vi "자판기.vi"() -> ()   [LabVIEW 2011]
panel:
  in  "거스름돈 반환":bool
  out "거스름돈":i32 format="%d \\"
  in  "투입금액":i32 format="%d \\"
  in  "생수":bool
  in  "사이다":bool
  in  "콜라":bool
  in  "커피":bool
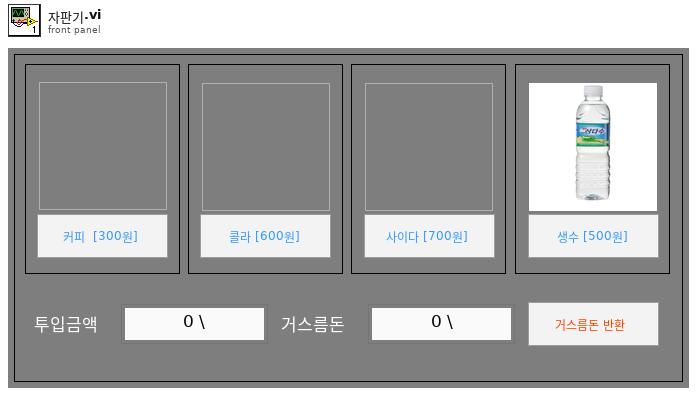
[diagram p1: front panel]
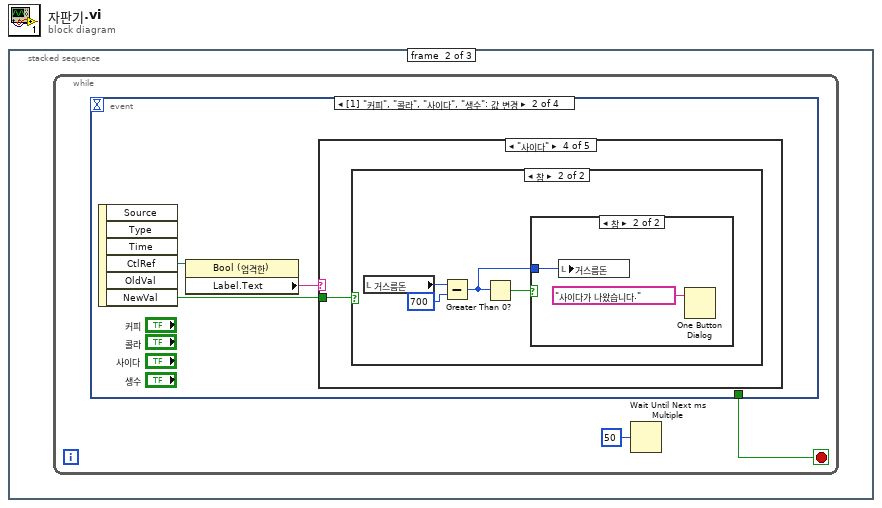
[diagram p0: block diagram]
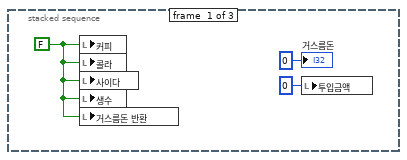
[diagram p2: hidden frame]
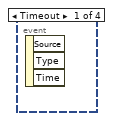
[diagram p3: hidden frame]
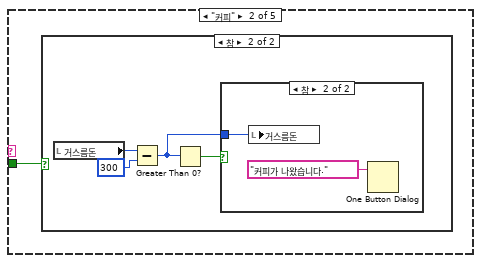
[diagram p5: hidden frame]
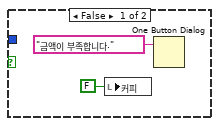
[diagram p7: hidden frame]
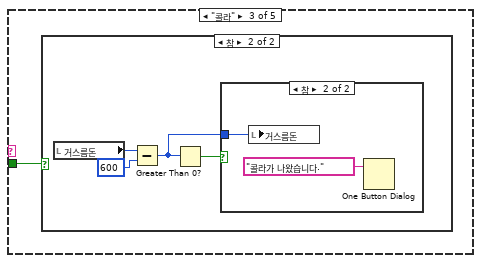
[diagram p8: hidden frame]
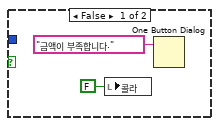
[diagram p10: hidden frame]
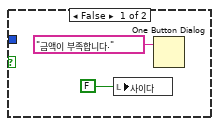
[diagram p12: hidden frame]
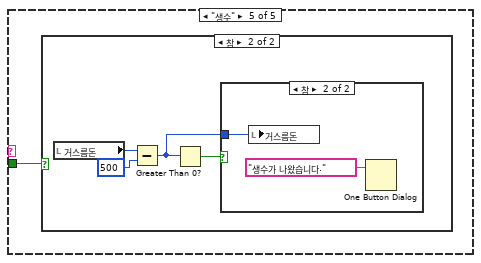
[diagram p13: hidden frame]
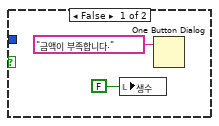
[diagram p15: hidden frame]
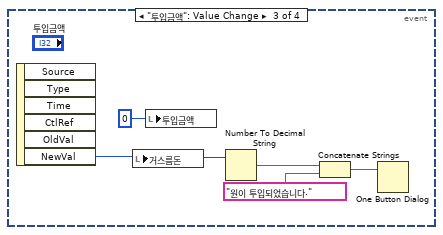
[diagram p16: hidden frame]
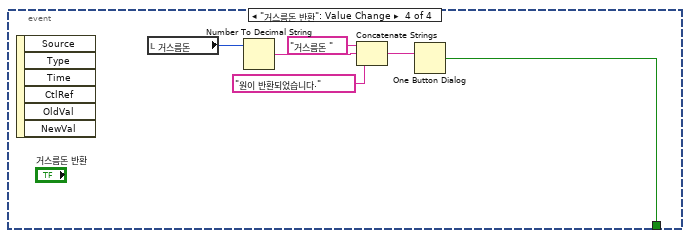
[diagram p17: hidden frame]
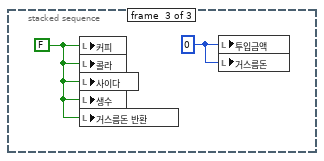
[diagram p18: hidden frame]
diagram:
  n1 = stacked-sequence {
    frame #0 {
      w3 = FALSE ("커피")
      n2 = local write "커피"(w3) -> ()
      n3 = local write "콜라"(w3) -> ()
      n4 = local write "사이다"(w3) -> ()
      n5 = local write "생수"(w3) -> ()
      n6 = local write "거스름돈 반환"(w3) -> ()
      n7 = local write "투입금액"(0 ("투입금액")) -> ()
      "거스름돈" <- 0 ("거스름돈")
    }
    frame #1 {
      n8 = while {
        stop <- w5 stop-if-true
        n9 = event shown="[1] \"커피\", \"콜라\", \"사이다\", \"생수\": 값 변경" {
          selector: _ -> [_ _ _ _]
          dyn-events: _ -> [_ _ _ _]
          timeout: _ -> [_ _ _ _]
          tunnel: [_ _ _ w50] -> w5
          event Timeout {
            n10 = event-data() -> ()  [unwired: 1 in, 3 out]
          }
          event "커피", "콜라", "사이다", "생수": Value Change {
            n11 = event-data() -> ("CtlRef"=w8:refnum<vi>, "NewVal"=w6:bool)  [unwired: 1 in, 4 out]
            n12 = property class="Bool (엄격한)"(reference=w8) -> ("Label.Text"=w7:string)  [unwired: 1 in, 2 out]
            n13 = case shown="\"사이다\"" w7 {
              tunnel: w6 -> [_ w9 w18 w27 w36]
              frame "거짓", Default {
              }
              frame "커피" {
                n14 = case shown="참" w9 {
                  frame False {
                  }
                  frame True {
                    n15 = local read "거스름돈"() -> (w11:i32)
                    n16 = Subtract(x=w11, y=300) -> (x-y=w10:i32)
                    n17 = Greater Than 0?(x=w10) -> (x > 0?=w12:bool)
                    n18 = case shown="참" w12 {
                      tunnel: w10 -> [_ w17]
                      frame False {
                        n19 = local write "커피"(FALSE ("커피")) -> ()
                        n20 = One Button Dialog(message="금액이 부족합니다." ("메시지")) -> ()  [unwired: 1 in, 1 out]
                      }
                      frame True {
                        n21 = local write "거스름돈"(w17) -> ()
                        n22 = One Button Dialog(message="커피가 나왔습니다." ("메시지")) -> ()  [unwired: 1 in, 1 out]
                      }
                    }
                  }
                }
              }
              frame "콜라" {
                n23 = case shown="참" w18 {
                  frame False {
                  }
                  frame True {
                    n24 = local read "거스름돈"() -> (w20:i32)
                    n25 = Subtract(x=w20, y=600) -> (x-y=w19:i32)
                    n26 = Greater Than 0?(x=w19) -> (x > 0?=w21:bool)
                    n27 = case shown="참" w21 {
                      tunnel: w19 -> [_ w26]
                      frame False {
                        n28 = local write "콜라"(FALSE ("커피")) -> ()
                        n29 = One Button Dialog(message="금액이 부족합니다." ("메시지")) -> ()  [unwired: 1 in, 1 out]
                      }
                      frame True {
                        n30 = local write "거스름돈"(w26) -> ()
                        n31 = One Button Dialog(message="콜라가 나왔습니다." ("메시지")) -> ()  [unwired: 1 in, 1 out]
                      }
                    }
                  }
                }
              }
              frame "사이다" {
                n32 = case shown="참" w27 {
                  frame False {
                  }
                  frame True {
                    n33 = local read "거스름돈"() -> (w29:i32)
                    n34 = Subtract(x=w29, y=700) -> (x-y=w28:i32)
                    n35 = Greater Than 0?(x=w28) -> (x > 0?=w30:bool)
                    n36 = case shown="참" w30 {
                      tunnel: w28 -> [_ w35]
                      frame False {
                        n37 = local write "사이다"(FALSE ("커피")) -> ()
                        n38 = One Button Dialog(message="금액이 부족합니다." ("메시지")) -> ()  [unwired: 1 in, 1 out]
                      }
                      frame True {
                        n39 = local write "거스름돈"(w35) -> ()
                        n40 = One Button Dialog(message="사이다가 나왔습니다." ("메시지")) -> ()  [unwired: 1 in, 1 out]
                      }
                    }
                  }
                }
              }
              frame "생수" {
                n41 = case shown="참" w36 {
                  frame False {
                  }
                  frame True {
                    n42 = local read "거스름돈"() -> (w38:i32)
                    n43 = Subtract(x=w38, y=500) -> (x-y=w37:i32)
                    n44 = Greater Than 0?(x=w37) -> (x > 0?=w39:bool)
                    n45 = case shown="참" w39 {
                      tunnel: w37 -> [_ w44]
                      frame False {
                        n46 = local write "생수"(FALSE ("커피")) -> ()
                        n47 = One Button Dialog(message="금액이 부족합니다." ("메시지")) -> ()  [unwired: 1 in, 1 out]
                      }
                      frame True {
                        n48 = local write "거스름돈"(w44) -> ()
                        n49 = One Button Dialog(message="생수가 나왔습니다." ("메시지")) -> ()  [unwired: 1 in, 1 out]
                      }
                    }
                  }
                }
              }
            }
          }
          event "투입금액": Value Change {
            n50 = event-data() -> ("NewVal"=w49:i32)  [unwired: 1 in, 5 out]
            n51 = local write "거스름돈"(w49) -> ()
            n52 = local write "투입금액"(0 ("투입금액")) -> ()
            n53 = Number To Decimal String(number=w49) -> (decimal integer string=w48:string)  [unwired: 1 in]
            n54 = Concatenate Strings(w48, "원이 투입되었습니다." ("문자열")) -> (w46:string)
            n55 = One Button Dialog(message=w46) -> ()  [unwired: 1 in, 1 out]
          }
          event "거스름돈 반환": Value Change {
            n56 = event-data() -> ()  [unwired: 1 in, 6 out]
            n57 = local read "거스름돈"() -> (w55:i32)
            n58 = Number To Decimal String(number=w55) -> (decimal integer string=w53:string)  [unwired: 1 in]
            n59 = Concatenate Strings("거스름돈 " ("문자열"), w53, "원이 반환되었습니다." ("문자열")) -> (w51:string)
            n60 = One Button Dialog(message=w51) -> (true=w50:bool)  [unwired: 1 in]
          }
        }
        n61 = Wait Until Next ms Multiple(millisecond multiple=u32 50 ("ms 배수")) -> ()  [unwired: 1 out]
      }
    }
    frame #2 {
      w57 = u64 0 ("투입금액")
      w56 = FALSE ("커피")
      n62 = local write "커피"(w56) -> ()
      n63 = local write "콜라"(w56) -> ()
      n64 = local write "사이다"(w56) -> ()
      n65 = local write "생수"(w56) -> ()
      n66 = local write "거스름돈 반환"(w56) -> ()
      n67 = local write "투입금액"(w57) -> ()
      n68 = local write "거스름돈"(w57) -> ()
    }
  }
